vi "Image To Tensor.vi"(8 "error in (no error)":errorcluster, 10 "Circle":T2, 11 "image data IN":T1) -> (0 "error out":errorcluster, 1 "image":picture, 2 "Data":sgl[](array[numeric]), 3 "image data OUT":T1)   [LabVIEW 2017, in "process_Angle.lvlib"]
doc: "Created IvanLis by LabVIEW Portal\nProfile: http://labviewportal.org/memberlist.php?mode=viewprofile&u=987\neMail: IvanLisanov@gMail.com\nTelegram: https://t.me/IvanLis"
uses:
  process_Angle.lvlib
  image_vi/image.lvlib
  process_YOLOv8/Circle.ctl
  process_YOLOv8/process_YOLOv8.lvlib
  <vilib>/picture/picture.llb/imagedata.ctl
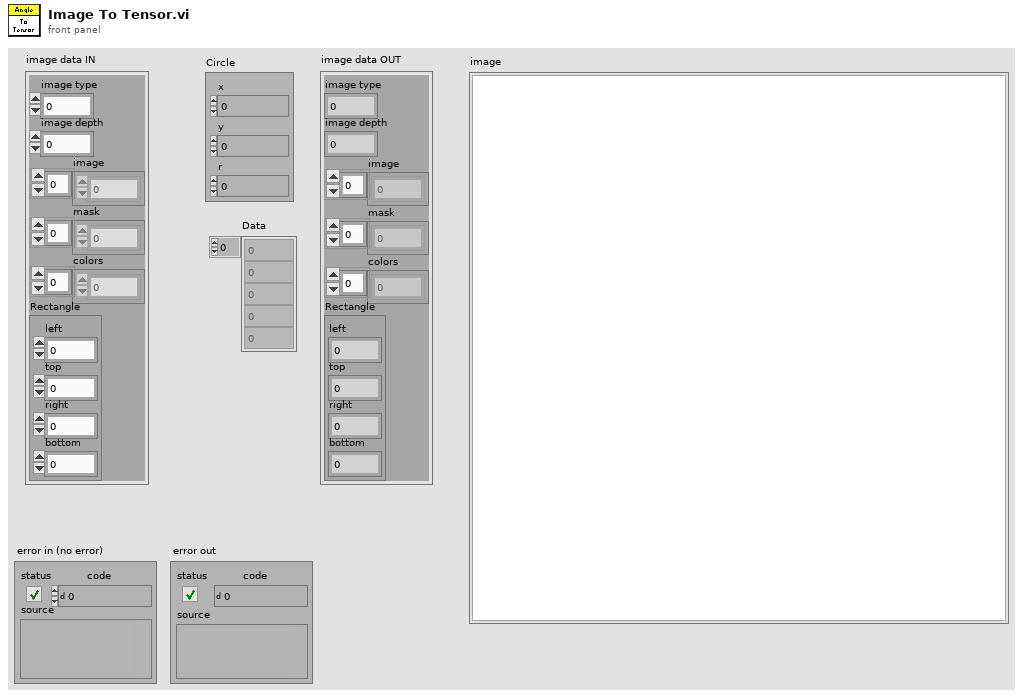
[diagram p1: front panel]
types:
  T1 = typedef "imagedata.ctl" = cluster{"image type":i32, "image depth":i32, "image":u8[], "mask":u8[], "colors":u32[], "Rectangle":cluster{"left":i16, "top":i16, "right":i16, "bottom":i16}}
  T2 = typedef "process_YOLOv8.lvlib/Circle.ctl" = cluster{"x":sgl, "y":sgl, "r":sgl}
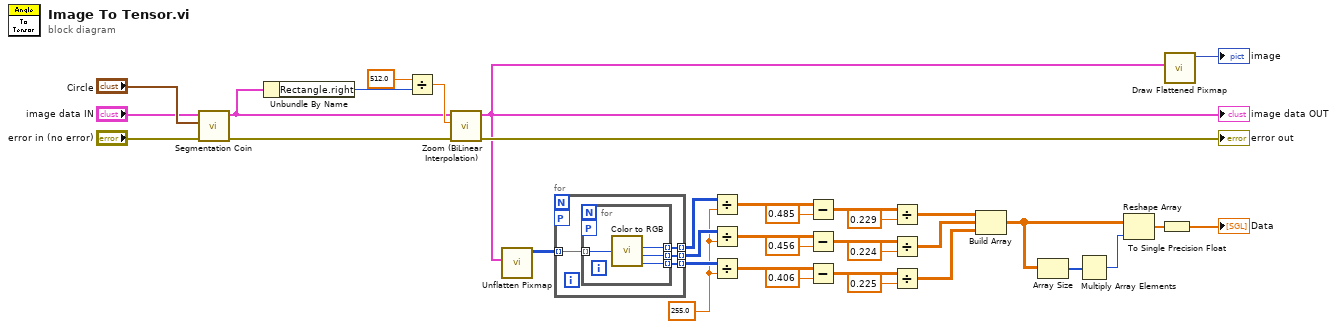
[diagram p0: block diagram]
diagram:
  w18 = 255.0 ("y")
  n1 = call "Segmentation Coin.vi"("error in (no error)"="error in (no error)", "Circle"="Circle", "image data in"="image data IN") -> ("error out"=w32:errorcluster, "image data out"=w33:T1)  [unwired: 7 in]
  n2 = Unbundle By Name(w33) -> ("Rectangle.right"=w34:i16)
  n3 = Divide(x=512.0, y=w34) -> (x/y=w36:dbl)
  n4 = call "Zoom (BiLinear Interpolation).vi"("error IN"=w32, "Zoom Coefficient"=w36, "image data IN"=w33) -> ("error OUT"=→"error out":errorcluster, "image data OUT"=w17:T1)  [unwired: 7 in]
  "image data OUT" <- w17
  n5 = call <vilib>:"Unflatten Pixmap.vi"("image data"=w17) -> ("24-bit pixmap"=w26:u32[][])  [unwired: 10 out]
  n6 = for {
    tunnel: w26 -> [w40] mode=indexing
    tunnel: [w39] -> w19 mode=indexing
    tunnel: [w38] -> w20 mode=indexing
    tunnel: [w37] -> w21 mode=indexing
    workers-P: _ -> [_]
    n7 = for {
      tunnel: w40 -> [w41] mode=indexing
      tunnel: [w44] -> w39 mode=indexing
      tunnel: [w43] -> w38 mode=indexing
      tunnel: [w42] -> w37 mode=indexing
      workers-P: _ -> [_]
      n8 = call <vilib>:"Color to RGB.vi"("Color"=w41) -> ("R"=w44:u8, "G"=w43:u8, "B"=w42:u8)  [unwired: 1 out]
    }
  }
  n9 = Divide(x=w19, y=w18) -> (x/y=w16:dbl[][])
  n10 = Divide(x=w20, y=w18) -> (x/y=w5:dbl[][])
  n11 = Divide(x=w21, y=w18) -> (x/y=w3:dbl[][])
  n12 = Subtract(x=w16, y=0.485) -> (x-y=w14:dbl[][])
  n13 = Subtract(x=w5, y=0.456) -> (x-y=w6:dbl[][])
  n14 = Subtract(x=w3, y=0.406) -> (x-y=w8:dbl[][])
  n15 = Divide(x=w14, y=0.229) -> (x/y=w13:dbl[][])
  n16 = Divide(x=w6, y=0.224) -> (x/y=w4:dbl[][])
  n17 = Divide(x=w8, y=0.225) -> (x/y=w2:dbl[][])
  n18 = Build Array(w13, w4, w2) -> (w23:dbl[][][])
  n19 = Array Size(array=w23) -> (size(s)=w22:i32[])
  n20 = Multiply Array Elements(1:w22) -> (0:w24:i32)
  n21 = Reshape Array(w23, w24) -> (w25:dbl[])
  n22 = To Single Precision Float(number=w25) -> (single precision float=→"Data":sgl[])
  n23 = call <vilib>:"Draw Flattened Pixmap.vi"("image data"=w17) -> ("new picture"=→"image":picture)  [unwired: 8 in]
